vi "WVFM.vi"(8 "dt":dbl, 10 "FPGA VI Reference In":refnum<k20>) -> (2 "VR array":waveform(sgl)[](array[waveform]), 3 "VL array":waveform(sgl)[](array[waveform]))   [LabVIEW 2016]
uses:
  <vilib>/Utility/error.llb/Error Cluster From Error Code.vi
  <vilib>/rvi/errors/niLvFpgaAdjustHostInterfaceError.vi
  <vilib>/rvi/interface/nirviReadWriteControl/nirviReadWriteControl.xnode
  NiFpgaLv.dll
  <vilib>/rvi/interface/Simulation/niFpgaSimulationCallBeginRW.vi
panel:
  in  "waveform":waveform(sgl)
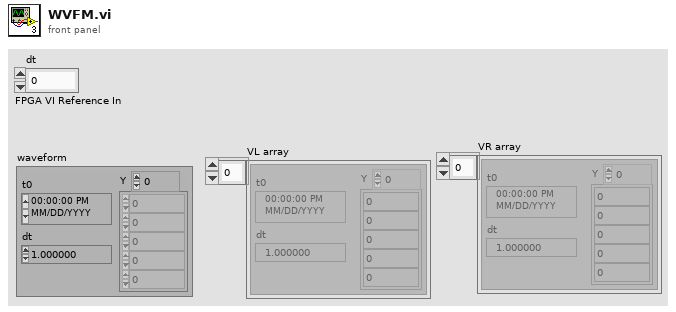
[diagram p1: front panel]
types:
  T1 = enum16{"Va L", "Vb L", "Vc L", "Ia", "Ib", "Ic", "Va R", "Vb R", "Vc R"}[]
  T2 = enum16{"Va L", "Vb L", "Vc L", "Ia", "Ib", "Ic", "Va R", "Vb R", "Vc R"}
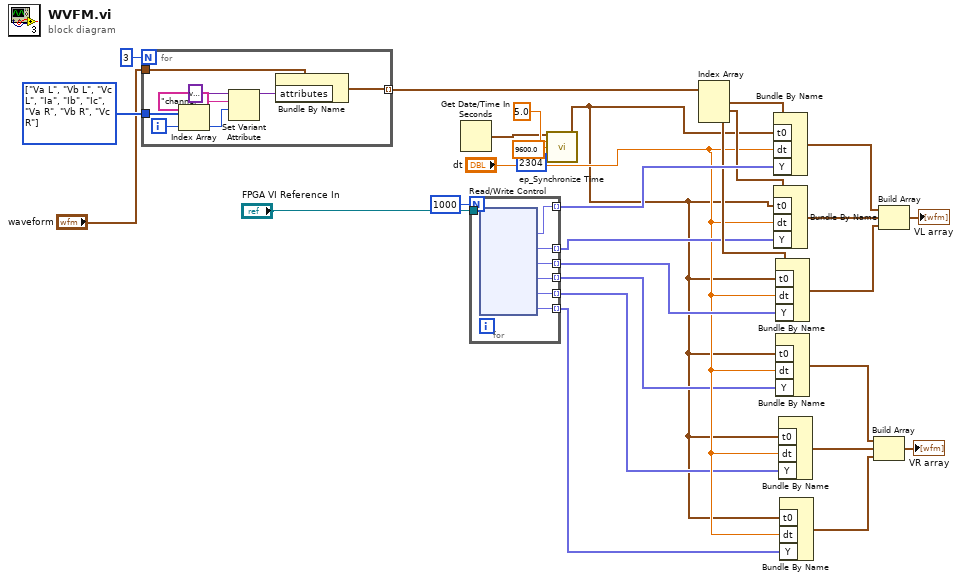
[diagram p0: block diagram]
diagram:
  w28 = T1 [enum."Va L", enum."Vb L", enum."Vc L", enum."Ia", enum."Ib", enum."Ic", enum."Va R", enum."Vb R", enum."Vc R"] items=["Va L", "Vb L", "Vc L", "Ia", "Ib", "Ic", "Va R", "Vb R", "Vc R"] ("Enum")
  n1 = for {
    N: 3 -> [_]
    tunnel: "waveform" -> [w32]
    tunnel: w28 -> [w35]
    tunnel: [w30] -> w27 mode=indexing
    i -> [w34]
    n2 = Index Array(array=w35, index=w34) -> (element=w33:T2)
    n3 = Set Variant Attribute(Variant=variant ("variant"), name="channel", value=w33) -> (Variant out=w31:variant)  [unwired: 1 in, 2 out]
    n4 = Bundle By Name(cluster=w32, "attributes"=w31) -> (w30:waveform(sgl))
  }
  n5 = Get Date/Time In Seconds() -> (seconds since 1Jan1904=w2:timestamp)
  n6 = for {
    N: 1000 -> [_]
    tunnel: "FPGA VI Reference In" -> [w44]
    tunnel: [w43] -> w23 mode=indexing
    tunnel: [w42] -> w19 mode=indexing
    tunnel: [w41] -> w20 mode=indexing
    tunnel: [w40] -> w9 mode=indexing
    tunnel: [w39] -> w8 mode=indexing
    tunnel: [w38] -> w7 mode=indexing
    n7 = xnode "Read/Write Control"("FPGA VI Reference In"=w44) -> ("V1L AB"=w43:fxp<+/-,26,5>, "V1L BC"=w42:fxp<+/-,26,5>, "V1L CA"=w41:fxp<+/-,26,5>, "V1R AB"=w40:fxp<+/-,26,5>, "V1R BC"=w39:fxp<+/-,26,5>, "V1R CA"=w38:fxp<+/-,12,5>)  [unwired: 1 in, 2 out]
  }
  n8 = call <vilib>:"ep_Synchronize Time.vi"("RT controler time in"=w2, "maximum time difference (sec)"=5.0, "sampling rate (Hz)"=9600.0, "basic calc. interval (samples)"=2304) -> ("RT controler time out"=w1:timestamp)  [unwired: 11 in]
  n9 = Index Array(array=w27) -> (element #1=w24:waveform(sgl), element #2=w22:waveform(sgl), element #3=w21:waveform(sgl))  [unwired: 3 in]
  n10 = Bundle By Name(cluster=w24, "t0"=w1, "dt"="dt", "Y"=w23) -> (w14:waveform(sgl))
  n11 = Bundle By Name(cluster=w22, "t0"=w1, "dt"="dt", "Y"=w19) -> (w13:waveform(sgl))
  n12 = Bundle By Name(cluster=w21, "t0"=w1, "dt"="dt", "Y"=w20) -> (w11:waveform(sgl))
  n13 = Bundle By Name("t0"=w1, "dt"="dt", "Y"=w9) -> (w6:waveform(sgl))  [unwired: 1 in]
  n14 = Bundle By Name("t0"=w1, "dt"="dt", "Y"=w8) -> (w5:waveform(sgl))  [unwired: 1 in]
  n15 = Bundle By Name("t0"=w1, "dt"="dt", "Y"=w7) -> (w4:waveform(sgl))  [unwired: 1 in]
  n16 = Build Array(w6, w5, w4) -> (→"VR array":waveform(sgl)[])
  n17 = Build Array(w14, w13, w11) -> (→"VL array":waveform(sgl)[])
